vi "USB-RS485_isol_Modbus_config.vi"(3 "Set RS-485 baud rate (bps)":u32, 4 "Action":string(combo)="E", 5 "Port":refnum<visa-resource-name>) -> (0 "Error Out":errorcluster, 1 "Returned RS-485 baud rate (bps)":u32, 2 "Returned error state":T1(ring))   [LabVIEW 2020]
doc: "Modbus RTU for Invertek drives. Paul Nathan 18-JUN-2022."
uses:
  <vilib>/Instr/_visa.llb/VISA Open Access Mode.ctl
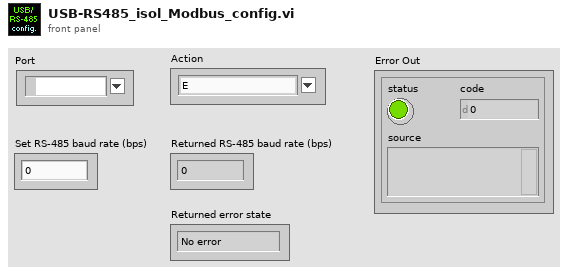
[diagram p1: front panel]
types:
  T1 = enum8{"No error", "Buffer overrun", "Bad checksum", "Bad frame"}
  T2 = typedef "VISA Open Access Mode.ctl" = u32
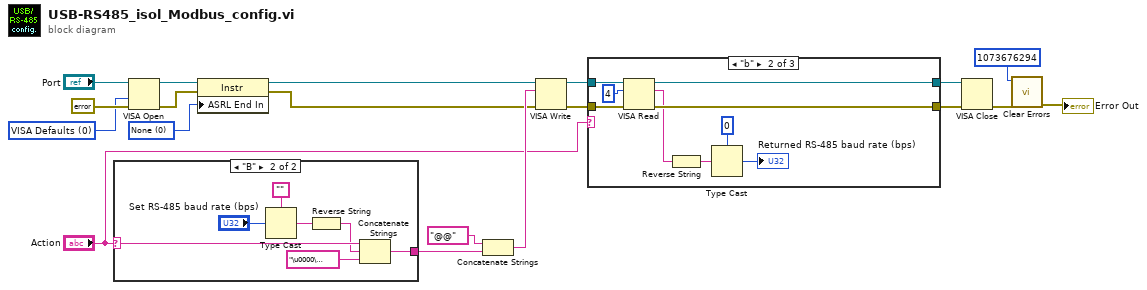
[diagram p0: block diagram]
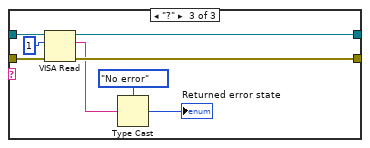
[diagram p3: hidden frame]
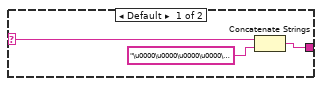
[diagram p4: hidden frame]
diagram:
  w18 = u16 0 items=["None", "Last Bit", "TermChar"] ("Serial Settings:End Mode for Reads")
  w16 = T2 0 items=["VISA Defaults"=0, "Exclusive Lock"=1, "Load Configured Settings"=4] ("Access Mode")
  n1 = case shown="\"B\"" "Action" {
    selector: "Action" -> [w21 w26]
    tunnel: [w22 w24] -> w7
    frame Default {
      n2 = Concatenate Strings(w21, "\u0000\u0000\u0000\u0000\u0000\u0000\u0000" ("string")) -> (w22:string)
    }
    frame "B" {
      n3 = Type Cast(type="", x="Set RS-485 baud rate (bps)") -> (*(type *) &x=w28:string)
      n4 = Reverse String(1:w28) -> (0:w25:string)
      n5 = Concatenate Strings(w26, w25, "\u0000\u0000\u0000" ("string")) -> (w24:string)
    }
  }
  n6 = VISA Open(access mode=w16, error in (no error)=errorcluster {"status"=FALSE, "code"=0, "source"=""}, VISA resource name="Port") -> (VISA resource name=w15:refnum<visa-resource-name>, error out=w14:errorcluster)  [unwired: 2 in]
  n7 = property class="Instr"(reference=w15, error in=w14, "ASRL End In"=w18) -> (reference out=w11:refnum<visa-resource-name>, error out=w10:errorcluster)
  n8 = Concatenate Strings("@@" ("string"), w7) -> (w12:string)
  n9 = VISA Write(VISA resource name=w11, write buffer=w12, error in (no error)=w10) -> (VISA resource name out=w9:refnum<visa-resource-name>, error out=w8:errorcluster)  [unwired: 1 out]
  n10 = case shown="\"b\"" "Action" {
    tunnel: w9 -> [w30 w39 w47]
    tunnel: w8 -> [w31 w38 w46]
    tunnel: [w31 w37 w45] -> w2
    tunnel: [w30 w36 w44] -> w3
    frame Default {
    }
    frame "b" {
      n11 = VISA Read(VISA resource name=w39, byte count=u32 4, error in (no error)=w38) -> (VISA resource name out=w36:refnum<visa-resource-name>, read buffer=w32:string, error out=w37:errorcluster)  [unwired: 1 out]
      n12 = Reverse String(1:w32) -> (0:w34:string)
      n13 = Type Cast(type=u32 0 ("byte count"), x=w34) -> (*(type *) &x=→"Returned RS-485 baud rate (bps)":u32)
    }
    frame "?" {
      n14 = VISA Read(VISA resource name=w47, byte count=u32 1, error in (no error)=w46) -> (VISA resource name out=w44:refnum<visa-resource-name>, read buffer=w41:string, error out=w45:errorcluster)  [unwired: 1 out]
      n15 = Type Cast(type=T1."No error" ("Returned error state"), x=w41) -> (*(type *) &x=→"Returned error state":T1)
    }
  }
  n16 = VISA Close(VISA resource name=w3, error in (no error)=w2) -> (error out=w6:errorcluster)
  n17 = call <vilib>:"Clear Errors.vi"("error in (no error)"=w6, "specific error code to clear (0: all)"=1073676294) -> ("error out"=→"Error Out":errorcluster)  [unwired: 4 in, 1 out]
